vi "Configure Trigger Out Amplitude.vi"(8 "error in (no error)":errorcluster, 10 "amplitude (1 V)":dbl=1.0 min=0.9 max=1.6, 11 "VISA resource name":refnum<visa-resource-name>) -> (0 "error out":errorcluster, 3 "VISA resource name out":refnum<visa-resource-name>)   [LabVIEW 2019, in "Pulse Rider PG-1000.lvlib"]
doc: "Sets the trigger output voltage level\n\nAmplitude: the amplitude in V, between 0.9 and 1.65"
uses:
  <instrlib>/Pulse Rider PG-1000/Pulse Rider PG-1000.lvlib
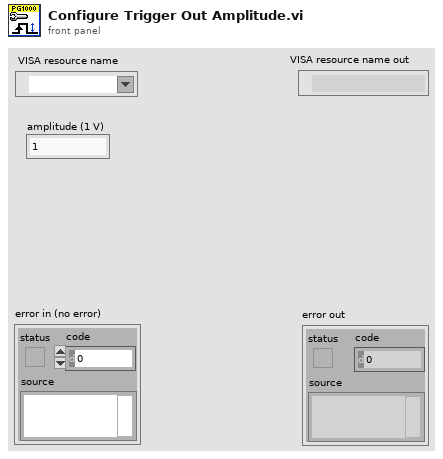
[diagram p1: front panel]
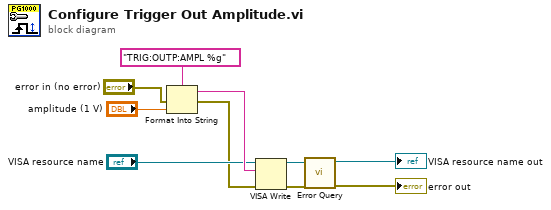
[diagram p0: block diagram]
diagram:
  n1 = Format Into String(format string="TRIG:OUTP:AMPL %g", error in="error in (no error)", "amplitude (1 V)") -> (resulting string=w7:string, error out=w1:errorcluster)  [unwired: 1 in]
  n2 = VISA Write(VISA resource name="VISA resource name", write buffer=w7, error in (no error)=w1) -> (VISA resource name out=w10:refnum<visa-resource-name>, error out=w9:errorcluster)  [unwired: 1 out]
  n3 = call <instrlib>:"Error Query.vi"("error in (no error)"=w9, "VISA resource name"=w10) -> ("error out"=→"error out":errorcluster, "VISA resource name out"=→"VISA resource name out":refnum<visa-resource-name>)  [unwired: 6 in, 2 out]
